vi "TestExec.Add User Docs from Local Config Dir.vi"(11 "Sys In":T1) -> (3 "Sys Out":T1)   [LabVIEW 2019]
uses:
  <vilib>/KATE/Module/Module Sys Info.ctl
  <vilib>/KATE/Config/Stored Controls/Class.SaveCtrls.lvclass
  <vilib>/KATE/Event Log/Event Notification/Event Notification.lvclass
  <vilib>/KATE/Config/App Data/Class.AppData.lvclass
  <vilib>/KATE/Subscription/Subscription.lvclass
  <vilib>/KATE/Queues/Q.Element.ctl
  <vilib>/KATE/Module/Module.SW Version Info.ctl
  <vilib>/KATE/Module/Module Config.ctl
  <vilib>/KATE/Module/Module.Working Dirs.ctl
  <vilib>/KATE/Files/File Utils.lvlib
  <vilib>/KATE/Menu/Menu Utils.lvlib
  <vilib>/KATE/Queues/Queue Utils.lvlib
  <vilib>/KATE/Module/Module Utils.lvlib
panel:
  # "Name, PN, Version, Note"
  # "Name, PN, Version, Note"
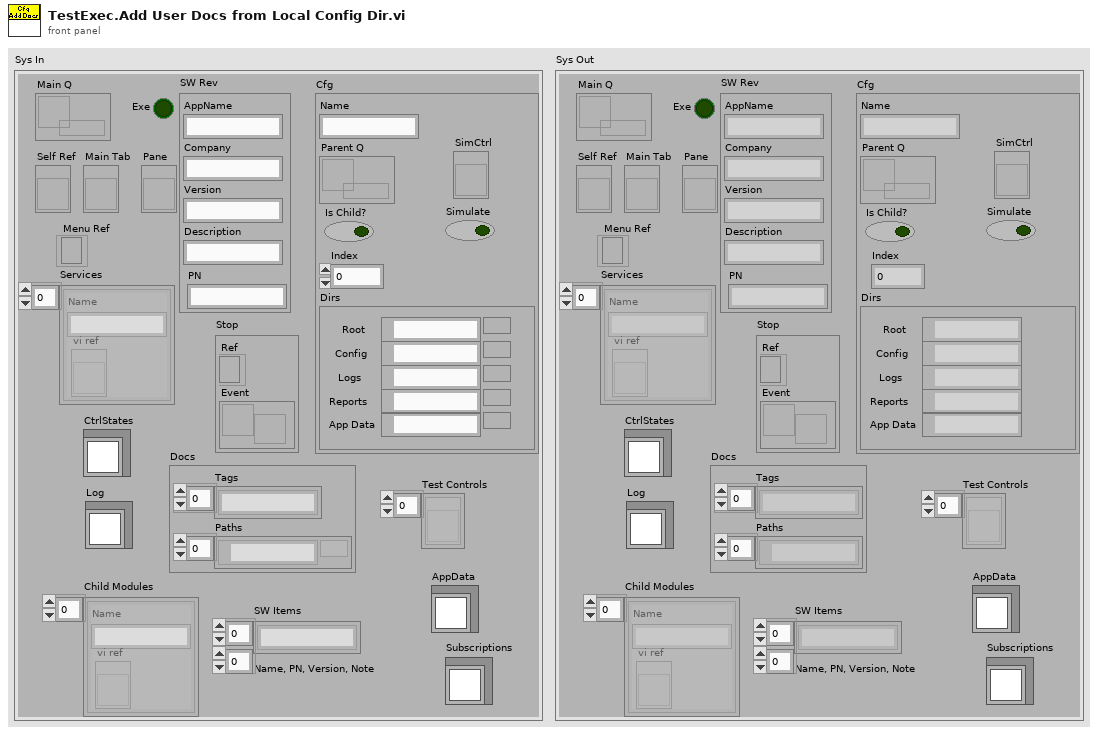
[diagram p1: front panel]
types:
  T1 = typedef "KATE_Lib.lvlib/Module Utils.lvlib/Module Sys Info.ctl" = cluster{"Main Q":refnum<queue>, "Exe":bool, "SW Rev":T2, "Self Ref":refnum<vi>, "Main Tab":refnum<vi>, "Pane":refnum<vi>, "Stop":cluster{"Ref":refnum<event-registration>, "Event":refnum<user-event>}, "Cfg":T3, "Services":cluster{"Name":string, "vi ref":refnum<vi>}[], "Menu Ref":refnum<k9>, "CtrlStates":refnum<class "Class.SaveCtrls.lvclass">, "Docs":cluster{"Tags":string[], "Paths":path[]}, "Log":refnum<class "Event Notification.lvclass">, "Test Controls":refnum<vi>[], "Child Modules":cluster{"Name":string, "vi ref":refnum<vi>}[], "SW Items":string[][], "AppData":refnum<class "Class.AppData.lvclass">, "Subscriptions":refnum<class "Subscription.lvclass">}
  T2 = typedef "KATE_Lib.lvlib/Module Utils.lvlib/Module.SW Version Info.ctl" = cluster{"AppName":string, "Company":string, "Version":string, "Description":string, "PN":string}
  T3 = typedef "KATE_Lib.lvlib/Module Utils.lvlib/Module Config.ctl" = cluster{"Name":string, "Parent Q":refnum<queue>, "Is Child?":bool, "Index":i32, "Dirs":T4, "Simulate":bool, "SimCtrl":refnum<vi>}
  T4 = typedef "KATE_Lib.lvlib/Module Utils.lvlib/Module.Working Dirs.ctl" = cluster{"Root":path, "Config":path, "Logs":path, "Reports":path, "App Data":path}
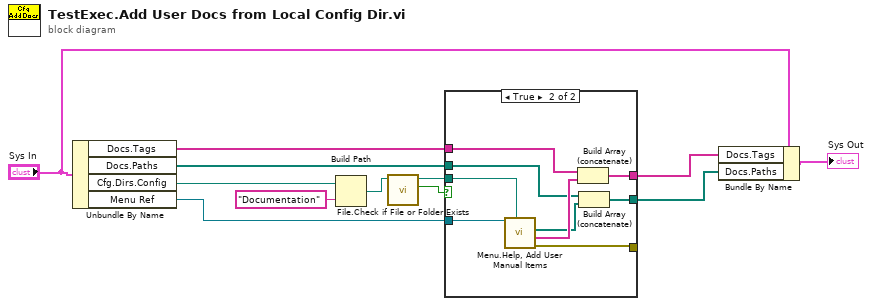
[diagram p0: block diagram]
diagram:
  n1 = Unbundle By Name("Sys In") -> ("Docs.Tags"=w7:string[], "Docs.Paths"=w6:path[], "Cfg.Dirs.Config"=w8:path, "Menu Ref"=w3:refnum<k9>)
  n2 = Build Path(base path=w8, name or relative path="Documentation") -> (appended path=w11:path)
  n3 = call <vilib>:"File.Check if File or Folder Exists.vi"("Path"=w11) -> ("Exists"=w9:bool, "Dup Path"=w10:path)  [unwired: 6 in, 3 out]
  n4 = case shown="True" w9 {
    tunnel: w3 -> [_ w23]
    tunnel: w10 -> [_ w22]
    tunnel: w7 -> [w14 w20]
    tunnel: w6 -> [w13 w19]
    tunnel: [w14 w17] -> w5
    tunnel: [w13 w16] -> w4
    tunnel: [_ w15] -> _
    frame False {
    }
    frame True {
      n5 = call <vilib>:"Menu.Help, Add User Manual Items.vi"("Doc Folder"=w22, "Menu Ref"=w23) -> ("error out"=w15:errorcluster, "Tags"=w21:string[], "Paths"=w18:path[])  [unwired: 6 in, 1 out]
      n6 = Build Array (concatenate)(w20, w21) -> (w17:string[])
      n7 = Build Array (concatenate)(w19, w18) -> (w16:path[])
    }
  }
  n8 = Bundle By Name(cluster="Sys In", "Docs.Tags"=w5, "Docs.Paths"=w4) -> (→"Sys Out":T1)
